vi "DSF.Shared.Configuration.Transfer.Check.Channel Parameters.Contiguous.vi"(8 "error in (no error)":errorcluster, 10 "Channel Descriptors in":T1[](array[typedef]) {"VS Channel Ref" format="%016x"; "Channel Parameters"."offset" format="%d bytes"}, 11 "Transfer Configuration in":refnum<class "DSF.Shared.Configuration.Transfer.lvclass">) -> (0 "error out":errorcluster, 2 "Channel Descriptors out":T1[](array[typedef]) {"VS Channel Ref" format="%016x"; "Channel Parameters"."offset" format="%d bytes"}, 3 "Transfer Configuration out":refnum<class "DSF.Shared.Configuration.Transfer.lvclass">)   [LabVIEW 2016, in "DSF.Shared.lvlib" / "DSF.Shared.Configuration.Transfer.lvclass"]
uses:
  DSF.Shared.Configuration.Transfer.lvclass
  Typedefs/DSF.Shared.Typedefs.Configuration.Transfer.Channel Descriptor.ctl
  Typedefs/DSF.Shared.Typedefs.Configuration.Transfer.Channel Parameters.ctl
  Typedefs/DSF.Shared.Typedefs.Data Type.ctl
  <vilib>/NI Veristand/Custom Device API/Custom Device Item Ref.ctl
  DSF.Shared.Configuration.Transfer.Errors.Channels Not Contiguous.vi
  <vilib>/NI Veristand/Custom Device API/Custom Device API.lvlib
  DSF.Shared.lvlib
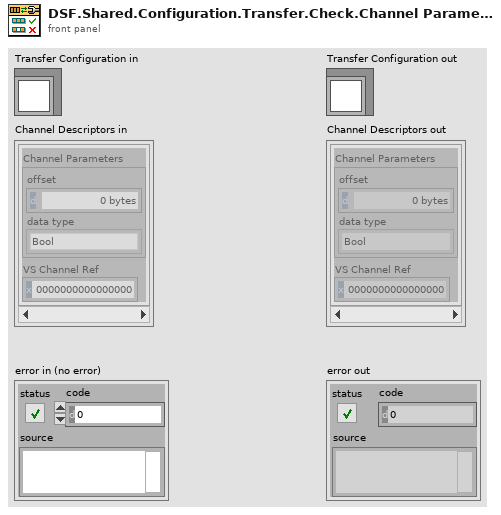
[diagram p1: front panel]
types:
  T1 = typedef "DSF.Shared.lvlib/DSF.Shared.Typedefs.Configuration.Transfer.Channel Descriptor.ctl" = cluster{"Channel Parameters":T2, "VS Channel Ref":T4}
  T2 = typedef "DSF.Shared.lvlib/DSF.Shared.Typedefs.Configuration.Transfer.Channel Parameters.ctl" = cluster{"offset":u64, "data type":T3}
  T3 = typedef "DSF.Shared.lvlib/DSF.Shared.Typedefs.Data Type.ctl" = enum8{"Bool", "SGL", "DBL", "I8", "I16", "I32", "I64", "U8", "U16", "U32", "U64"}
  T4 = typedef "Custom Device API.lvlib/Custom Device Item Ref.ctl" = u64
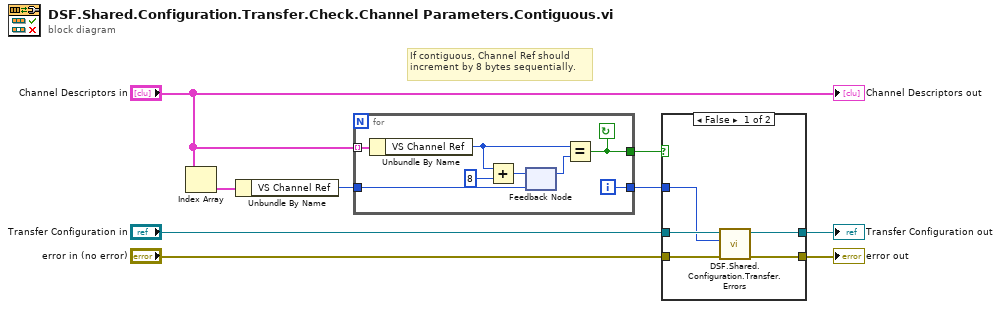
[diagram p0: block diagram]
diagram:
  # "If contiguous, Channel Ref should increment by 8 bytes sequentially."
  n1 = Index Array(array="Channel Descriptors in") -> (element=w9:T1)  [unwired: 1 in]
  n2 = Unbundle By Name(w9) -> ("VS Channel Ref"=w8:T4)
  n3 = for {
    tunnel: "Channel Descriptors in" -> [w17] mode=indexing
    tunnel: w8 -> [w15]
    tunnel: [w11] -> w2
    tunnel: [w10] -> w1
    i -> [w11]
    stop <- w10 continue-if-true
    n4 = Unbundle By Name(w17) -> ("VS Channel Ref"=w14:T4)
    n5 = Add(x=w14, y=T4 8) -> (x+y=w16:T4)
    n6 = feedback #1(w15) -> (w13:T4)
    n7 = feedback-in #1(w16) -> ()
    n8 = Equal?(x=w14, y=w13) -> (x = y?=w10:bool)
  }
  n9 = case shown="False" w1 {
    tunnel: [w22 w23] -> w6
    tunnel: "error in (no error)" -> [w21 w23]
    tunnel: "Transfer Configuration in" -> [w20 w24]
    tunnel: [w19 w24] -> w3
    tunnel: w2 -> [w18 _]
    frame False {
      n10 = call-poly "DSF.Shared.Configuration.Transfer.Errors.vi"("error in (no error)"=w21, "bad descriptor index"=w18, "Transfer Configuration in"=w20) -> ("error out"=w22:errorcluster, "Transfer Configuration out"=w19:refnum<class "DSF.Shared.Configuration.Transfer.lvclass">)  [unwired: 7 in]
    }
    frame True {
    }
  }
  "error out" <- w6
  "Transfer Configuration out" <- w3
  "Channel Descriptors out" <- "Channel Descriptors in"
